vi "CodeConvert(SubVI).vi"(1 "Code":string) -> (0 "Code_array":dbl[](array[numeric]))   [LabVIEW 2017]
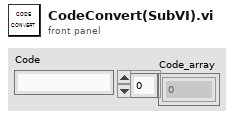
[diagram p1: front panel]
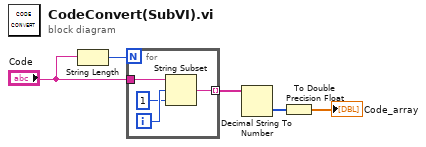
[diagram p0: block diagram]
diagram:
  n1 = String Length(string="Code") -> (length=w5:i32)
  n2 = for {
    N: w5 -> [_]
    tunnel: "Code" -> [w9]
    tunnel: [w7] -> w4 mode=indexing
    i -> [w8]
    n3 = String Subset(string=w9, offset (0)=w8, length (rest)=1 ("길이(나머지)")) -> (substring=w7:string)
  }
  n4 = Decimal String To Number(string=w4) -> (number=w2:i32[])  [unwired: 2 in, 1 out]
  n5 = To Double Precision Float(number=w2) -> (double precision float=→"Code_array":dbl[])
